vi "init.vi"(8 "error in (no error)":errorcluster caption="entrée d'erreur (pas d'erreur)", 9 "json of params":string, 10 "import":string, 11 "Model en entrée":refnum<class "Model.lvclass">) -> (0 "error out":errorcluster caption="sortie d'erreur", 3 "Model en sortie":refnum<class "Model.lvclass">)   [LabVIEW 2020, in "Model.lvclass"]
doc: "Initialize the model in the python session.\n\nYou can specify the import command: from sklearn.linear_model import LogisticRegression.\nYou can pass the parameters of the model in JSON format."
uses:
  Model.lvclass
  C:/Users/cipop/TDF Dropbox/2_Technologies de France/1 - Services et Etudes/PLAIY/2 - DEV/PLAIYLAB/code/Python/Python.lvclass
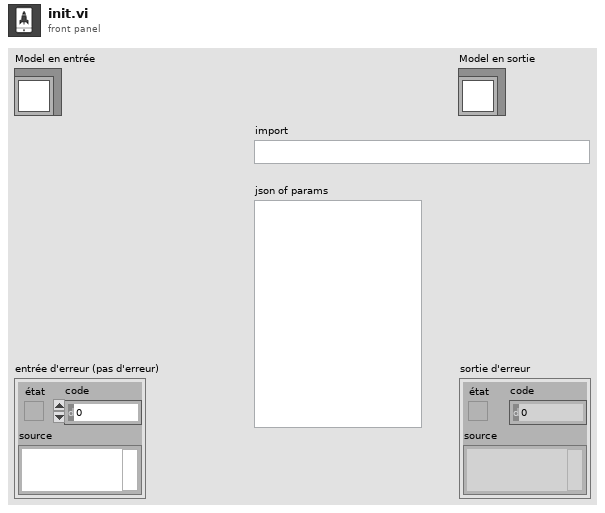
[diagram p1: front panel]
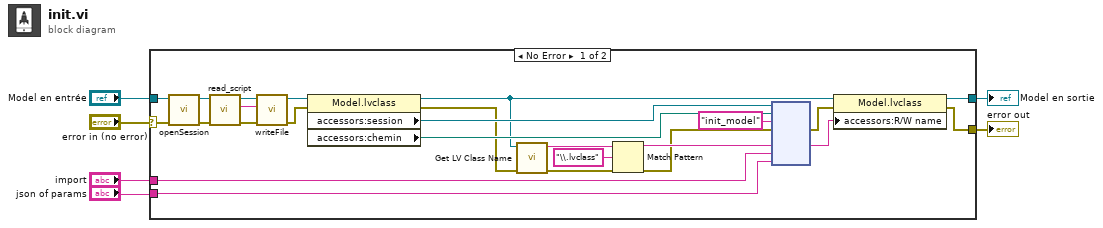
[diagram p0: block diagram]
diagram:
  n1 = case shown="No Error" "error in (no error)" {
    selector: "error in (no error)" -> [w29 w32]
    tunnel: [w12 w32] -> w5
    tunnel: [w11 w31] -> w3
    tunnel: "Model en entrée" -> [w30 w31]
    tunnel: "json of params" -> [w7 _]
    tunnel: "import" -> [w8 _]
    frame No Error {
      n2 = call-dynamic "openSession.vi"("error in (no error)"=w29, "Python en entrée"=w30) -> ("error out"=w9:errorcluster, "Python en sortie"=w10:refnum<class "Model.lvclass">)  [unwired: 8 in]
      n3 = call-dynamic "read_script.vi"("error in (no error)"=w9, "Model en entrée"=w10) -> ("error out"=w26:errorcluster, "script"=w27:string, "Model en sortie"=w28:refnum<class "Model.lvclass">)  [unwired: 7 in]
      n4 = call-dynamic "writeFile.vi"("error in (no error)"=w26, "script"=w27, "Python en entrée"=w28) -> ("error out"=w23:errorcluster, "Python en sortie"=w24:refnum<class "Model.lvclass">)  [unwired: 7 in]
      n5 = property class="Model.lvclass"(reference=w24, error in=w23) -> (reference out=w15:refnum<class "Model.lvclass">, error out=w17:errorcluster, "accessors:session"=w22:refnum<k35>, "accessors:chemin"=w21:path)
      n6 = call <vilib>:"Get LV Class Name.vi"("error in (no error)"=w17, "object"=w15) -> ("error out"=w16:errorcluster, "class name"=w20:string)  [unwired: 8 in]
      n7 = Match Pattern(string=w20, regular expression="\\.lvclass") -> (before substring=w18:string)  [unwired: 1 in, 3 out]
      n8 = node(w22, w21, "init_model" ("nom de la fonction"), w16, w18, w8, w7) -> (w13:errorcluster, w14:string)  [unwired: 4 in, 3 out]
      n9 = property class="Model.lvclass"(reference=w15, error in=w13, "accessors:R/W name"=w14) -> (reference out=w11:refnum<class "Model.lvclass">, error out=w12:errorcluster)
    }
    frame Error {
    }
  }
  "error out" <- w5
  "Model en sortie" <- w3
